vi "Module Identities.vi"(8 "error in (no error)":errorcluster, 11 "HTTP Manager in":refnum<class "HTTP Manager.lvclass">) -> (0 "error out":errorcluster, 2 "Identities":refnum<class "Identity.lvclass">[](array[class]), 3 "HTTP Manager out":refnum<class "HTTP Manager.lvclass">)   [LabVIEW 2020, in "Volatus.lvlib" / "HTTP Manager.lvclass"]
uses:
  HTTP Manager.lvclass
  Identity/Identity.lvclass
  HTTP Manager.lvclass/HTTP Manager.ctl
  HTTP Manager Identity/HTTP Manager Identity.lvclass
  C:/dev/lv20CE/relink/lv-volatus/Volatus/HTTP Manager Identity/HTTP Manager Identity.lvclass
  C:/dev/lv20CE/relink/lv-volatus/Volatus/Identity/Identity.lvclass
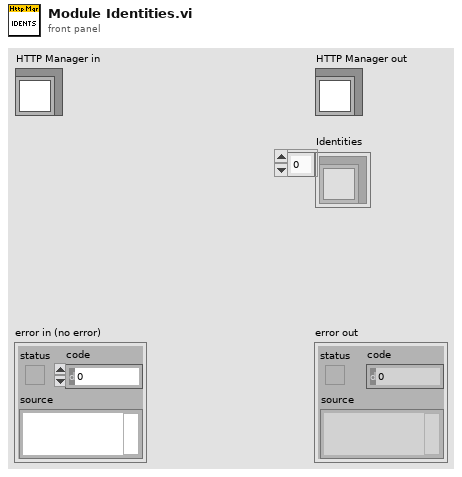
[diagram p1: front panel]
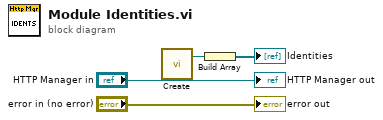
[diagram p0: block diagram]
diagram:
  n1 = call "Create.vi"() -> ("HTTP Manager Identity out"=w2:refnum<class "HTTP Manager Identity.lvclass">)  [unwired: 7 in]
  n2 = Build Array(w2) -> (→"Identities":refnum<class "HTTP Manager Identity.lvclass">[])
  "error out" <- "error in (no error)"
  "HTTP Manager out" <- "HTTP Manager in"
